vi "leebinario_LACECAL.vi"() -> ()   [LabVIEW 2015]
panel:
  out "Lectura de acelerómetros y wheel sensors":waveform(sgl)[](graph)
  in  "Folder Path":path
  out "error out":errorcluster
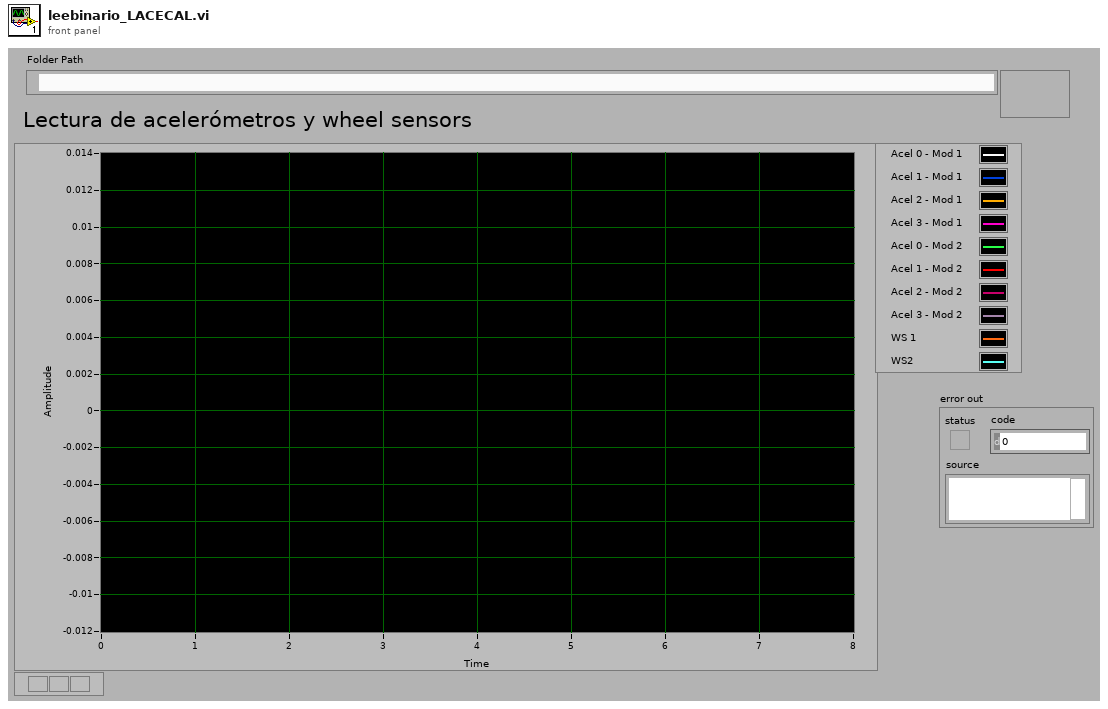
[diagram p1: front panel]
types:
  T1 = enum16{"big-endian, network order", "native, host order", "little-endian"}
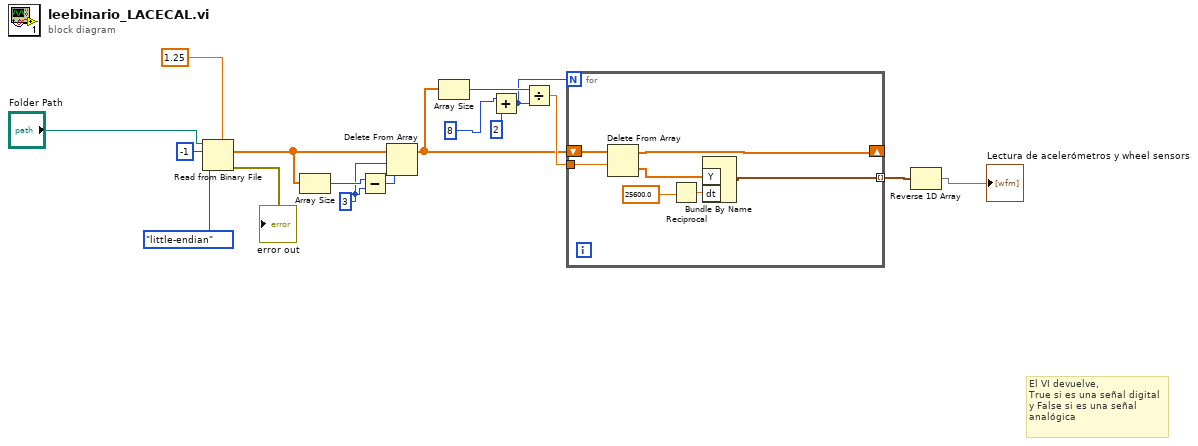
[diagram p0: block diagram]
diagram:
  w11 = 3 ("length")
  # "El VI devuelve,\nTrue si es una señal digital\ny False si es una señal\nanalógica"
  n1 = Read from Binary File(5:sgl 1.25, 9:T1."little-endian" ("byte order (0:big-endian, network order)"), 10:-1 ("count (1)"), 11:"Folder Path") -> (0:→"error out":errorcluster, 2:w10:sgl[])  [unwired: 1 in, 3 out]
  n2 = Array Size(array=w10) -> (size(s)=w13:i32)
  n3 = Subtract(x=w13, y=w11) -> (x-y=w12:i32)
  n4 = Delete From Array(array=w10, length=w11, index=w12) -> (array with subset deleted=w7:sgl[])  [unwired: 1 out]
  n5 = Array Size(array=w7) -> (size(s)=w9:i32)
  n6 = Add(x=8 ("y"), y=2) -> (x+y=w4:i32)
  n7 = Divide(x=w9, y=w4) -> (x/y=w8:dbl)
  n8 = for {
    N: w4 -> [_]
    tunnel: [w24] -> w3 mode=indexing
    shift-right: [w20] -> _
    shift-left: w7 -> [w21]
    tunnel: w8 -> [w19]
    n9 = Delete From Array(array=w21, length=w19) -> (deleted portion=w18:sgl[], array with subset deleted=w20:sgl[])  [unwired: 1 in]
    n10 = Reciprocal(x=25600.0 ("dt")) -> (1/x=w22:dbl)
    n11 = Bundle By Name("Y"=w18, "dt"=w22) -> (w24:waveform(sgl))  [unwired: 1 in]
  }
  n12 = Reverse 1D Array(array=w3) -> (reversed array=→"Lectura de acelerómetros y wheel sensors":waveform(sgl)[])
